vi "Scanner_01.vi"() -> ()   [LabVIEW 2011]
panel:
  out "Position":dbl[](array[numeric])
  out "String":string
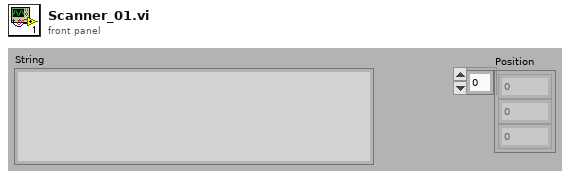
[diagram p1: front panel]
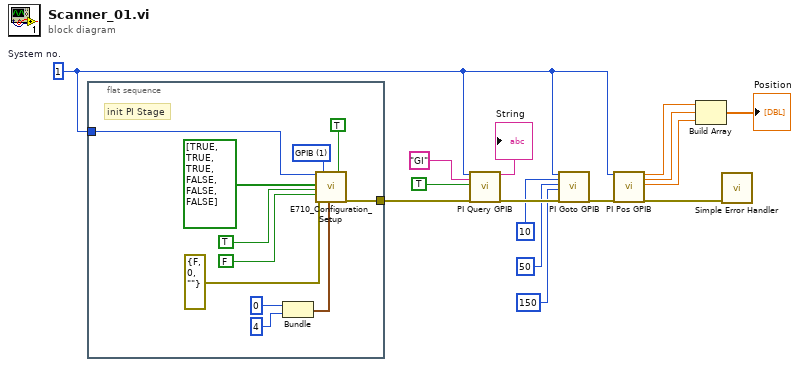
[diagram p0: block diagram]
diagram:
  w4 = 1  # System no.
  n1 = flat-sequence {
    tunnel: [w21] -> w15
    tunnel: w4 -> [w20]
    frame #0 {
      w23 = u16 1 items=["RS232", "GPIB"] ("Interface")
      # "init PI Stage"
      n2 = Bundle(0, 4) -> (w18:cluster{i32, i32})  [unwired: 1 out]
      n3 = call "E710_Configuration_Setup.vi"("System no."=w20, "Are stages connected?"=bool[] [TRUE, TRUE, TRUE, FALSE, FALSE, FALSE], "Change servo \nstatus to ON?"=TRUE ("Change servo \nstatus to ON?"), "Perform autozero?"=FALSE ("All axes?"), "error in"=errorcluster {"status"=FALSE, "code"=0, "source"=""}, "Interface"=w23, "GPIB settings"=w18, "Move to middle?"=TRUE) -> ("error out"=w21:errorcluster)  [unwired: 4 in, 7 out]
    }
  }
  n4 = call "PI Query GPIB.vi"("System no."=w4, "String to send"="GI", "Attach Linefeed?"=TRUE, "error in"=w15) -> ("String read"=→"String":string, "error out"=w5:errorcluster)  [unwired: 13 in, 1 out]
  n5 = call "PI Goto GPIB.vi"("System no."=w4, "x-position"=10, "y-position"=50, "z-position"=150, "error in"=w5) -> ("error out"=w6:errorcluster)  [unwired: 14 in]
  n6 = call "PI Pos GPIB.vi"("System no."=w4, "error in"=w6) -> ("x-position"=w8:dbl, "y-position"=w9:dbl, "z-position"=w7:dbl, "error out"=w11:errorcluster)  [unwired: 14 in]
  n7 = Build Array(w8, w9, w7) -> (→"Position":dbl[])
  n8 = call <vilib>:"Simple Error Handler.vi"("error in (no error)"=w11) -> ()  [unwired: 4 in, 5 out]
